vi "Balance_fb.vi"(8 "error in (no error)":errorcluster, 10 "Balance":string, 11 "ATM-Controller in":refnum<class "ATM-Controller.lvclass">) -> (0 "error out":errorcluster, 3 "ATM-Controller out":refnum<class "ATM-Controller.lvclass">)   [LabVIEW 2025, in "ATM-Controller.lvlib" / "ATM-Controller.lvclass"]
uses:
  ATM-Controller.lvclass
  ATM-Controller.lvclass/ATM-Controller.ctl
  DisplayConsole Messages/Update_Status_Display Msg/Update_Status_Display Msg.lvclass
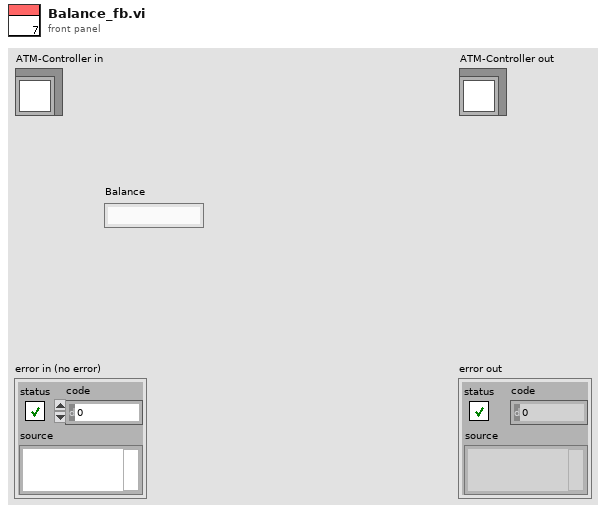
[diagram p1: front panel]
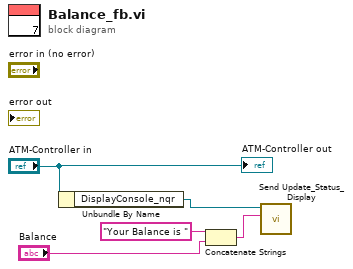
[diagram p0: block diagram]
diagram:
  n1 = Unbundle By Name("ATM-Controller in") -> ("DisplayConsole_nqr"=w4:refnum<class "Message Enqueuer.lvclass">)
  n2 = Concatenate Strings("Your Balance is ", "Balance") -> (w1:string)
  n3 = call "Send Update_Status_Display.vi"("Status"=w1, "Message Enqueuer"=w4) -> ()  [unwired: 8 in, 2 out]
  "ATM-Controller out" <- "ATM-Controller in"
